vi "Write Events.vi"(10 "Events":refnum<user-event>[](array[refnum]), 11 "Samples in":refnum<class "Samples.lvclass">) -> (3 "Samples out":refnum<class "Samples.lvclass">)   [LabVIEW 2015, in "AMS UI.lvlib" / "Samples.lvclass"]
uses:
  Samples.lvclass
  Samples.lvclass/Samples.ctl
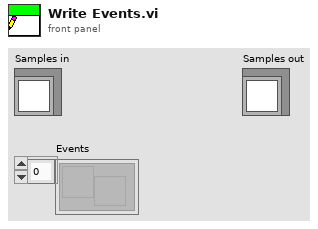
[diagram p1: front panel]
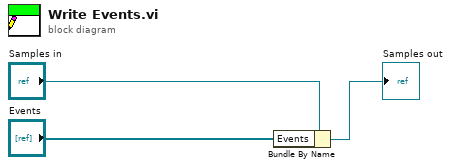
[diagram p0: block diagram]
diagram:
  n1 = Bundle By Name(cluster="Samples in", "Events"="Events") -> (→"Samples out":refnum<class "Samples.lvclass">)
